vi "Create Function with Line Number.vi"(0 "Script Lines in":string[](array[string]), 11 "error in (no error)":errorcluster) -> (4 "Functions":T1[](array[typedef]), 15 "error out":errorcluster)   [LabVIEW 2019]
uses:
  Line Details.ctl
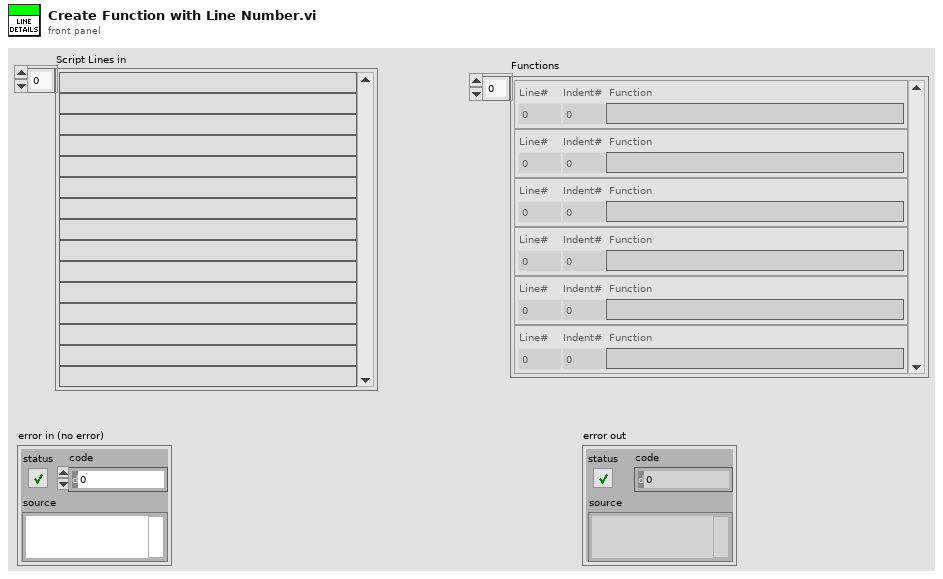
[diagram p1: front panel]
types:
  T1 = typedef "Line Details.ctl" = cluster{"Line#":i64, "Indent#":i64, "Function":string}
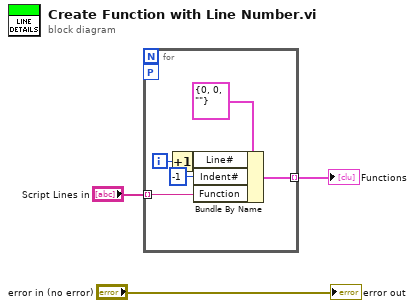
[diagram p0: block diagram]
diagram:
  n1 = for {
    tunnel: "Script Lines in" -> [w8] mode=indexing
    tunnel: [w5] -> w1 mode=indexing
    workers-P: _ -> [_]
    i -> [w7]
    n2 = Increment(x=w7) -> (x+1=w4:i32)
    n3 = Bundle By Name(cluster=T1 {"Line#"=0, "Indent#"=0, "Function"=""} ("Function Details"), "Line#"=w4, "Indent#"=i64 -1, "Function"=w8) -> (w5:T1)
  }
  "Functions" <- w1
  "error out" <- "error in (no error)"
